vi "世界-自动读取D盘根目录txt中的数据设置相机位姿.vi"() -> ()   [LabVIEW 2012]
uses:
  <vilib>/picture/3D Picture Control/NI_3D Picture Control.lvlib
panel:
  out "相机坐标":cluster{"x":dbl, "y":dbl, "z":dbl}
  in  "旋转轴1":cluster{"X":sgl, "Y":sgl, "Z":sgl}={"X"=1.0, "Y"=0.0, "Z"=0.0}
  in  "旋转轴2":cluster{"X":sgl, "Y":sgl, "Z":sgl}={"X"=0.0, "Y"=1.0, "Z"=0.0}
  in  "旋转轴3":cluster{"X":sgl, "Y":sgl, "Z":sgl}={"X"=0.0, "Y"=0.0, "Z"=1.0}
  out "3D重绘":refnum<vi>(3d-picture)
  in  "停止":bool
  out "第三次旋转":sgl caption="角"
  out "第二次旋转":sgl caption="角"
  out "第一次旋转":sgl caption="角"
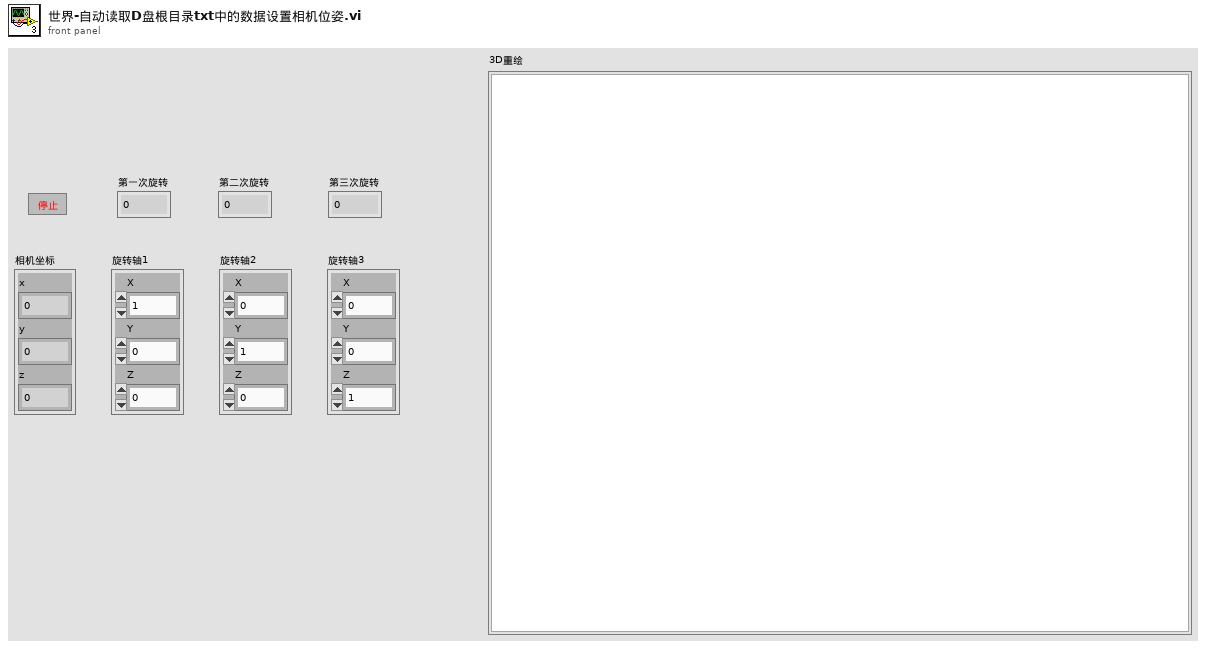
[diagram p1: front panel]
types:
  T1 = cluster{"Red":sgl, "Green":sgl, "Blue":sgl, "Alpha":sgl}
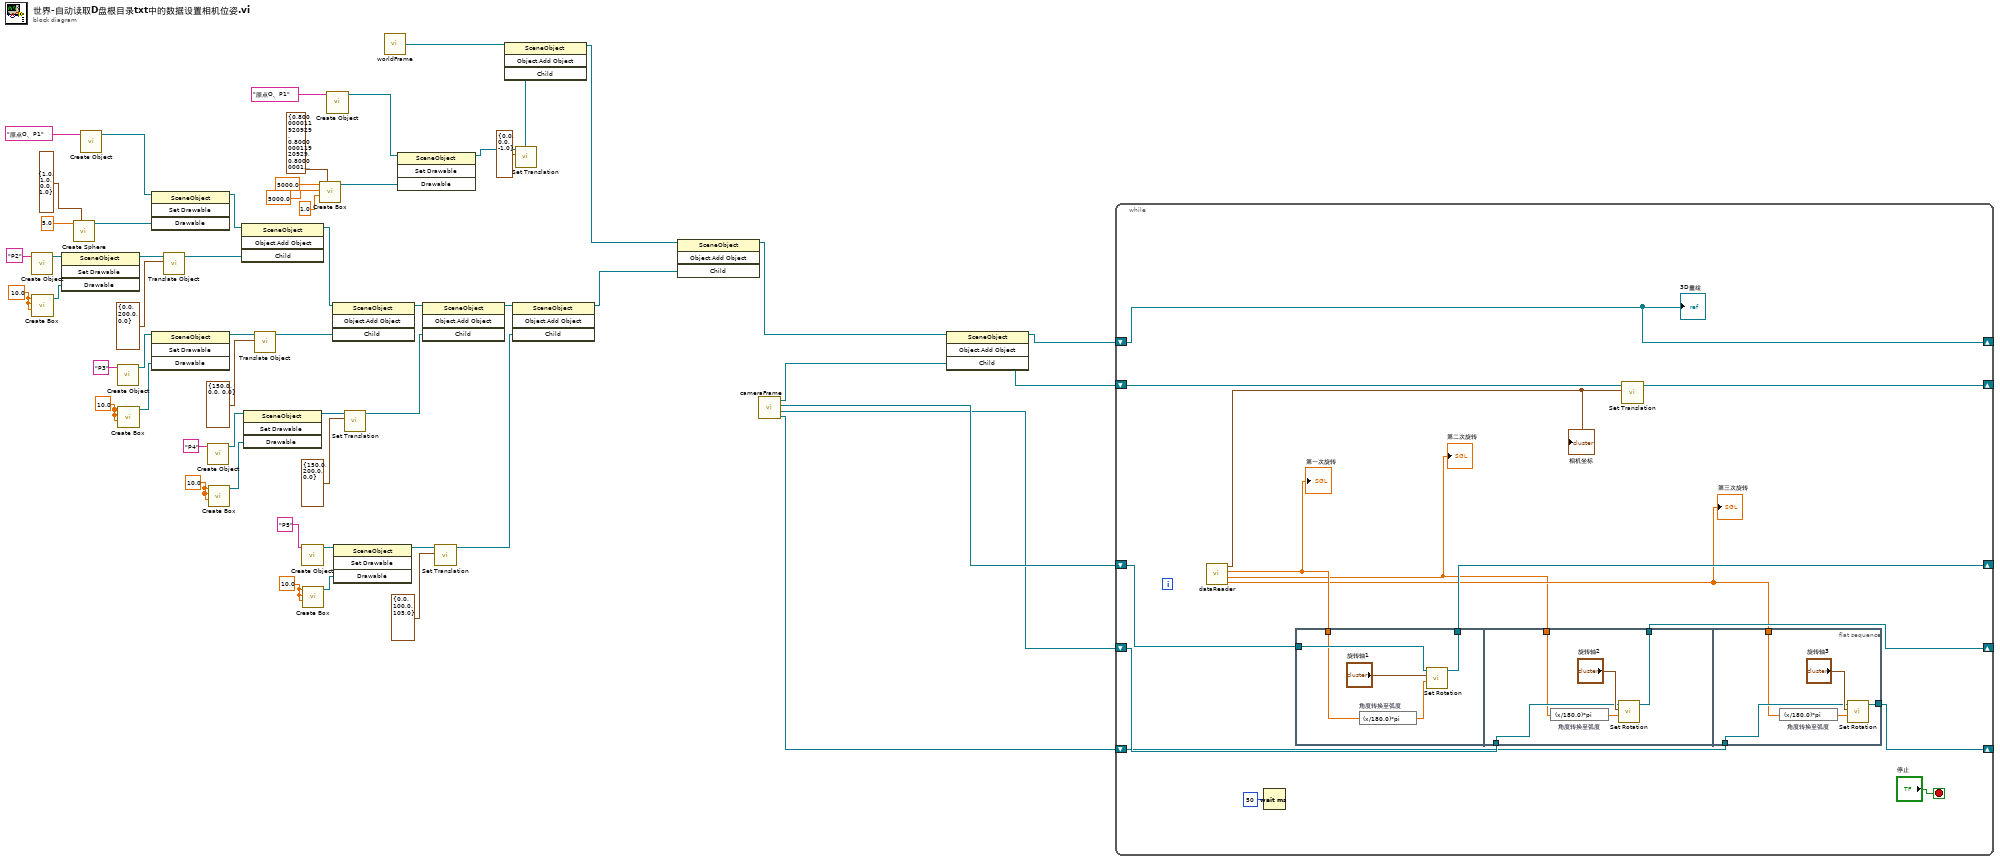
[diagram p0: block diagram]
diagram:
  w25 = sgl 10.0 ("Length X")
  w38 = sgl 10.0 ("Length X")
  w50 = sgl 10.0 ("Length X")
  w44 = sgl 10.0 ("Length X")
  n1 = call <vilib>:"Create Object.vi"("Name"="P2") -> ("Scene:New Object"=w42:refnum<vi>)  [unwired: 9 in, 1 out]
  n2 = call <vilib>:"Create Box.vi"("Length Z"=w44, "Length Y"=w44, "Length X"=w44) -> ("New Box Refnum"=w43:refnum<vi>)  [unwired: 7 in, 1 out]
  n3 = invoke class="SceneObject" method="Set Drawable"(reference=w42, "Drawable"=w43) -> (reference out=w45:refnum<vi>)  [unwired: 2 in, 3 out]
  n4 = call <vilib>:"Create Sphere.vi"("Color"=T1 {"Red"=1.0, "Green"=1.0, "Blue"=0.0, "Alpha"=1.0}, "Radius"=sgl 5.0 ("Length X")) -> ("New Sphere Refnum"=w41:refnum<vi>)  [unwired: 8 in, 1 out]
  n5 = call <vilib>:"Create Object.vi"("Name"="原点O、P1") -> ("Scene:New Object"=w40:refnum<vi>)  [unwired: 9 in, 1 out]
  n6 = call <vilib>:"Create Object.vi"("Name"="P3") -> ("Scene:New Object"=w47:refnum<vi>)  [unwired: 9 in, 1 out]
  n7 = call <vilib>:"Create Box.vi"("Length Z"=w50, "Length Y"=w50, "Length X"=w50) -> ("New Box Refnum"=w51:refnum<vi>)  [unwired: 7 in, 1 out]
  n8 = invoke class="SceneObject" method="Set Drawable"(reference=w40, "Drawable"=w41) -> (reference out=w18:refnum<vi>)  [unwired: 2 in, 3 out]
  n9 = invoke class="SceneObject" method="Set Drawable"(reference=w47, "Drawable"=w51) -> (reference out=w48:refnum<vi>)  [unwired: 2 in, 3 out]
  n10 = call <vilib>:"Translate Object.vi"("Translation"=cluster{"X":sgl, "Y":sgl, "Z":sgl} {"X"=0.0, "Y"=200.0, "Z"=0.0}, "Scene.Object In"=w45) -> ("Scene.Object Out"=w17:refnum<vi>)  [unwired: 8 in, 1 out]
  n11 = call <vilib>:"Create Object.vi"("Name"="P4") -> ("Scene:New Object"=w35:refnum<vi>)  [unwired: 9 in, 1 out]
  n12 = call <vilib>:"Create Box.vi"("Length Z"=w38, "Length Y"=w38, "Length X"=w38) -> ("New Box Refnum"=w39:refnum<vi>)  [unwired: 7 in, 1 out]
  n13 = invoke class="SceneObject" method="Object.Add Object"(reference=w18, "Child"=w17) -> (reference out=w16:refnum<vi>)  [unwired: 2 in, 3 out]
  n14 = invoke class="SceneObject" method="Set Drawable"(reference=w35, "Drawable"=w39) -> (reference out=w36:refnum<vi>)  [unwired: 2 in, 3 out]
  n15 = call <vilib>:"Translate Object.vi"("Translation"=cluster{"X":sgl, "Y":sgl, "Z":sgl} {"X"=150.0, "Y"=0.0, "Z"=0.0}, "Scene.Object In"=w48) -> ("Scene.Object Out"=w52:refnum<vi>)  [unwired: 8 in, 1 out]
  n16 = call <vilib>:"Create Object.vi"("Name"="P5") -> ("Scene:New Object"=w22:refnum<vi>)  [unwired: 9 in, 1 out]
  n17 = call <vilib>:"Create Box.vi"("Length Z"=w25, "Length Y"=w25, "Length X"=w25) -> ("New Box Refnum"=w26:refnum<vi>)  [unwired: 7 in, 1 out]
  n18 = call <vilib>:"Create Box.vi"("Color"=T1 {"Red"=0.8, "Green"=0.8, "Blue"=0.8, "Alpha"=0.2}, "Length Z"=sgl 1.0, "Length Y"=sgl 5000.0, "Length X"=sgl 5000.0) -> ("New Box Refnum"=w13:refnum<vi>)  [unwired: 6 in, 1 out]
  n19 = call <vilib>:"Create Object.vi"("Name"="原点O、P1") -> ("Scene:New Object"=w12:refnum<vi>)  [unwired: 9 in, 1 out]
  n20 = invoke class="SceneObject" method="Object.Add Object"(reference=w16, "Child"=w52) -> (reference out=w33:refnum<vi>)  [unwired: 2 in, 3 out]
  n21 = invoke class="SceneObject" method="Set Drawable"(reference=w22, "Drawable"=w26) -> (reference out=w23:refnum<vi>)  [unwired: 2 in, 3 out]
  n22 = call <vilib>:"Set Translation.vi"("Translation"=cluster{"X":sgl, "Y":sgl, "Z":sgl} {"X"=150.0, "Y"=200.0, "Z"=0.0}, "Scene Object"=w36) -> ("Translated Object"=w34:refnum<vi>)  [unwired: 8 in, 1 out]
  n23 = call "worldFrame.vi"() -> ("引用输出"=w6:refnum<vi>)
  n24 = invoke class="SceneObject" method="Set Drawable"(reference=w12, "Drawable"=w13) -> (reference out=w4:refnum<vi>)  [unwired: 2 in, 3 out]
  n25 = invoke class="SceneObject" method="Object.Add Object"(reference=w33, "Child"=w34) -> (reference out=w20:refnum<vi>)  [unwired: 2 in, 3 out]
  n26 = call <vilib>:"Set Translation.vi"("Translation"=cluster{"X":sgl, "Y":sgl, "Z":sgl} {"X"=0.0, "Y"=100.0, "Z"=105.0}, "Scene Object"=w23) -> ("Translated Object"=w19:refnum<vi>)  [unwired: 8 in, 1 out]
  n27 = invoke class="SceneObject" method="Object.Add Object"(reference=w20, "Child"=w19) -> (reference out=w15:refnum<vi>)  [unwired: 2 in, 3 out]
  n28 = call <vilib>:"Set Translation.vi"("Translation"=cluster{"X":sgl, "Y":sgl, "Z":sgl} {"X"=0.0, "Y"=0.0, "Z"=-1.0}, "Scene Object"=w4) -> ("Translated Object"=w3:refnum<vi>)  [unwired: 8 in, 1 out]
  n29 = invoke class="SceneObject" method="Object.Add Object"(reference=w6, "Child"=w3) -> (reference out=w5:refnum<vi>)  [unwired: 2 in, 3 out]
  n30 = invoke class="SceneObject" method="Object.Add Object"(reference=w5, "Child"=w15) -> (reference out=w14:refnum<vi>)  [unwired: 2 in, 3 out]
  n31 = call "cameraFrame.vi"() -> ("x轴旋转引用"=w55:refnum<vi>, "y轴旋转引用"=w56:refnum<vi>, "z轴旋转引用"=w57:refnum<vi>, "相机引用"=w54:refnum<vi>)
  n32 = invoke class="SceneObject" method="Object.Add Object"(reference=w14, "Child"=w54) -> (reference out=w1:refnum<vi>, "Child"=w53:refnum<vi>)  [unwired: 2 in, 2 out]
  n33 = while {
    shift-right: [w66] -> _
    shift-left: w55 -> [w67]
    shift-right: [w65] -> _
    shift-left: w56 -> [w68]
    shift-right: [w64] -> _
    shift-left: w57 -> [w69]
    shift-right: [w71] -> _
    shift-left: w53 -> [w70]
    shift-right: [w63] -> _
    shift-left: w1 -> [w63]
    stop <- "停止" stop-if-true
    n34 = call "dataReader.vi"() -> ("thetaz"=w60:dbl, "thetay"=w59:dbl, "thetax"=w61:dbl, "平移"=w62:cluster{"数值":dbl, "数值 2":dbl, "数值 3":dbl})
    "第一次旋转" <- w61
    "第二次旋转" <- w59
    "第三次旋转" <- w60
    "相机坐标" <- w62
    n35 = Wait (ms)(milliseconds to wait=u32 50 ("等待时间（毫秒）")) -> ()  [unwired: 1 out]
    n36 = flat-sequence {
      tunnel: w69 -> [w75]
      tunnel: [w74] -> w64
      tunnel: w61 -> [w73]
      tunnel: w68 -> [w80]
      tunnel: [w79] -> w65
      tunnel: w59 -> [w78]
      tunnel: w67 -> [w85]
      tunnel: [w84] -> w66
      tunnel: w60 -> [w83]
      frame #0 {
        n37 = expression code="(x/180.0)*pi" "角度转换至弧度"(w73) -> (w77:dbl)
        n38 = call <vilib>:"Set Rotation.vi"("Angle"=w77, "Axis"="旋转轴1", "Scene Object"=w75) -> ("Rotated Scene Object"=w74:refnum<vi>)  [unwired: 7 in, 1 out]
      }
      frame #1 {
        n39 = expression code="(x/180.0)*pi" "角度转换至弧度"(w78) -> (w82:dbl)
        n40 = call <vilib>:"Set Rotation.vi"("Angle"=w82, "Axis"="旋转轴2", "Scene Object"=w80) -> ("Rotated Scene Object"=w79:refnum<vi>)  [unwired: 7 in, 1 out]
      }
      frame #2 {
        n41 = expression code="(x/180.0)*pi" "角度转换至弧度"(w83) -> (w87:dbl)
        n42 = call <vilib>:"Set Rotation.vi"("Angle"=w87, "Axis"="旋转轴3", "Scene Object"=w85) -> ("Rotated Scene Object"=w84:refnum<vi>)  [unwired: 7 in, 1 out]
      }
    }
    n43 = call <vilib>:"Set Translation.vi"("Translation"=w62, "Scene Object"=w70) -> ("Translated Object"=w71:refnum<vi>)  [unwired: 8 in, 1 out]
    "3D重绘" <- w63
  }
